vi "Ultrasonic Flip Flop.vi"(10 "Distance":dbl) -> (2 "output":bool)   [LabVIEW 2011]
uses:
  <vilib>/functionblocks/Bistables/SR Bistable/SR Bistable.vi
  <vilib>/functionblocks/FB Core/FB Core.xnode
  <vilib>/functionblocks/NI_FunctionBlock Libraries.lvlib
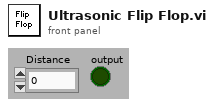
[diagram p1: front panel]
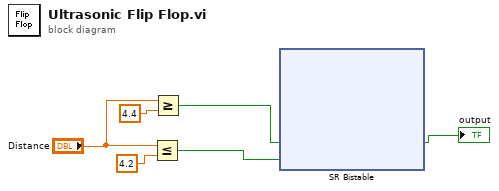
[diagram p0: block diagram]
diagram:
  n1 = Less Or Equal?(x="Distance", y=4.2) -> (x <= y?=w6:bool)
  n2 = Greater Or Equal?(x="Distance", y=4.4) -> (x >= y?=w2:bool)
  n3 = xnode "SR Bistable"("reset"=w2, "set"=w6) -> ("output"=→"output":bool)  [unwired: 1 in, 1 out]
